vi "Get Row and Colum (SubVI).vi"(8 "Dim":u32=256, 10 "Colum In":u32, 11 "Row In":u32) -> (0 "Last Pixel?":bool, 2 "Colum Out":u32, 3 "Row Out":u32, 4 "Pixel B":u32, 6 "Pixel A":u32)   [LabVIEW 2017]
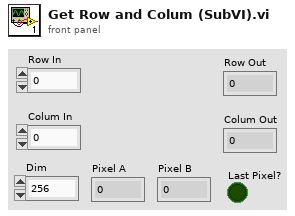
[diagram p1: front panel]
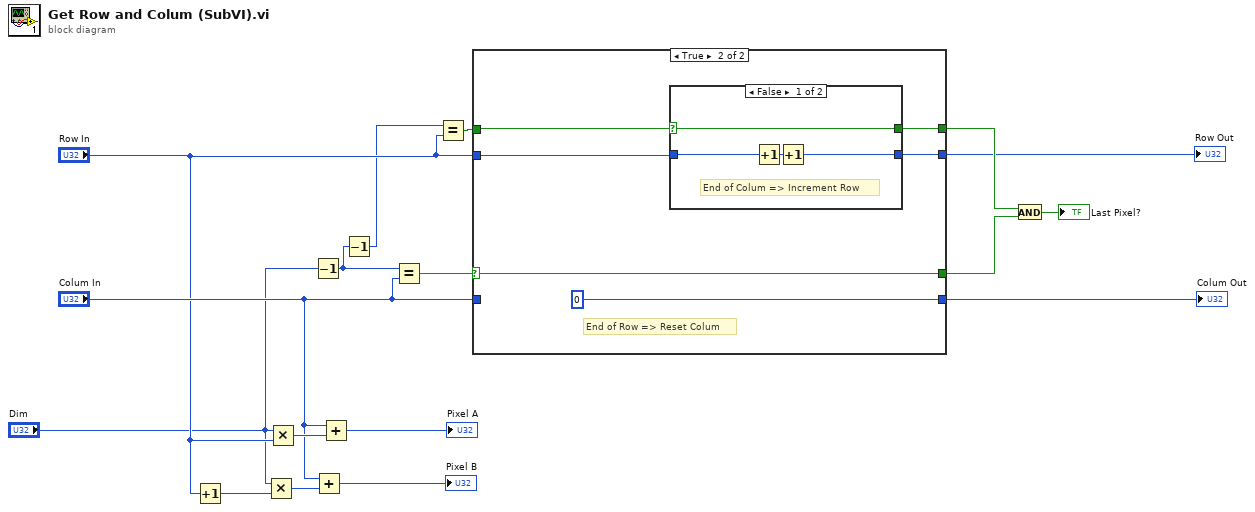
[diagram p0: block diagram]
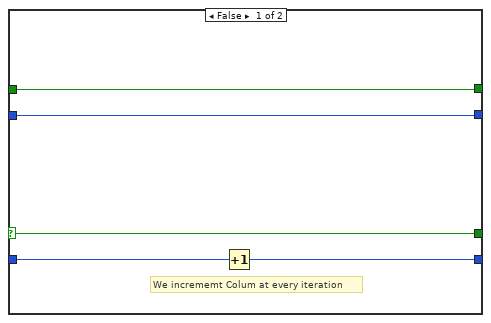
[diagram p2: hidden frame]
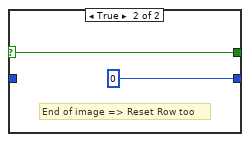
[diagram p3: hidden frame]
diagram:
  n1 = Increment(x="Row In") -> (x+1=w17:u32)
  n2 = Multiply(x="Dim", y=w17) -> (x*y=w16:u32)
  n3 = Multiply(x="Dim", y="Row In") -> (x*y=w10:u32)
  n4 = Decrement(x="Dim") -> (x-1=w2:u32)
  n5 = Add(x="Colum In", y=w16) -> (x+y=→"Pixel B":u32)
  n6 = Add(x="Colum In", y=w10) -> (x+y=→"Pixel A":u32)
  n7 = Decrement(x=w2) -> (x-1=w1:u32)
  n8 = Equal?(x=w2, y="Colum In") -> (x = y?=w15:bool)
  n9 = Equal?(x=w1, y="Row In") -> (x = y?=w7:bool)
  n10 = case shown="True" w15 {
    selector: w15 -> [w20 w27]
    tunnel: [w22 u32 0] -> w14
    tunnel: "Colum In" -> [w21 _]
    tunnel: [w20 w27] -> w13
    tunnel: w7 -> [w18 w26]
    tunnel: "Row In" -> [w19 w23]
    tunnel: [w19 w25] -> w4
    tunnel: [w18 w24] -> w6
    frame False {
      # "We incrememt Colum at every iteration"
      n11 = Increment(x=w21) -> (x+1=w22:u32)
    }
    frame True {
      # "End of Row => Reset Colum"
      n12 = case shown="False" w26 {
        selector: w26 -> [w29 w33]
        tunnel: [w30 u32 0] -> w25
        tunnel: w23 -> [w31 _]
        tunnel: [w29 w33] -> w24
        frame False {
          # "End of Colum => Increment Row"
          n13 = Increment(x=w31) -> (x+1=w32:u32)
          n14 = Increment(x=w32) -> (x+1=w30:u32)
        }
        frame True {
          # "End of image => Reset Row too"
        }
      }
    }
  }
  "Row Out" <- w4
  "Colum Out" <- w14
  n15 = And(x=w6, y=w13) -> (x .and. y?=→"Last Pixel?":bool)
